vi "Ordenar_Trama.vi"(6 "offset (0) 3":i32, 7 "offset (0) 4":i32, 9 "offset (0) 2":i32, 10 "offset (0) 1":i32, 11 "format string":string) -> (3 "String":string)   [LabVIEW 2017]
doc: "Subvi que ordena valores de la trama recibida de arduino"
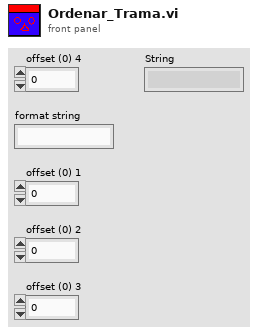
[diagram p1: front panel]
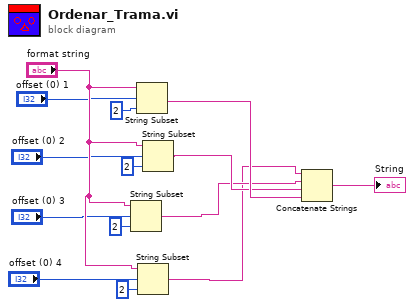
[diagram p0: block diagram]
diagram:
  n1 = String Subset(string="format string", offset (0)="offset (0) 3", length (rest)=2 ("length (rest)")) -> (substring=w11:string)
  n2 = String Subset(string="format string", offset (0)="offset (0) 1", length (rest)=2 ("length (rest)")) -> (substring=w13:string)
  n3 = String Subset(string="format string", offset (0)="offset (0) 4", length (rest)=2 ("length (rest)")) -> (substring=w10:string)
  n4 = String Subset(string="format string", offset (0)="offset (0) 2", length (rest)=2 ("length (rest)")) -> (substring=w12:string)
  n5 = Concatenate Strings(w10, w11, w12, w13) -> (→"String":string)
